vi "DDS_Clock.vi"() -> ()   [LabVIEW 2016] (continued)
dcp wait:1h:\rdcp wait::DROVER\rdcp 0 spi:DRL=0x4DD2F1AA4DC5D639\rdcp 0 spi:DRSS=0x1E1FFFFFFFF\rdcp 0 spi:DRR=0x70000\rdcp 0 update:+d\rdcp 0 update:-d\rdcp wait:1h:\rdcp wait::DROVER\rdcp 0 spi:DRL=0x4DC5D6394DB8BAC7\rdcp 0 spi:DRSS=0x1E1FFFFFFFF\rdcp 0 spi:DRR=0x70000\rdcp 0 update:+d\rdcp 0 update:-d\rdcp wait:1h:\rdcp wait::DROVER\rdcp 0 spi:DRL=0x4DB8BAC74DAB9F56\rdcp 0 spi:DRSS=0x1E1FFFFFFFF\rdcp 0 spi:DRR=0x70000\rdcp 0 update:+d\rdcp 0 update:-d\rdcp wait:1h:\rdcp wait::DROVER\rdcp 0 spi:DRL=0x4DAB9F564D9E83E4\rdcp 0 spi:DRSS=0x1E1FFFFFFFF\rdcp 0 spi:DRR=0x70000\rdcp 0 update:+d\rdcp 0 update:-d\rdcp wait:1h:\rdcp wait::DROVER\rdcp 0 spi:DRL=0x4D9E83E44D916873\rdcp 0 spi:DRSS=0x1E1FFFFFFFF\rdcp 0 spi:DRR=0x70000\rdcp 0 update:+d\rdcp 0 update:-d\rdcp wait:1h:\rdcp wait::DROVER\rdcp 0 spi:DRL=0x4D9168734D844D01\rdcp 0 spi:DRSS=0x1E1FFFFFFFF\rdcp 0 spi:DRR=0x70000\rdcp 0 update:+d\rdcp 0 update:-d\rdcp wait:1h:\rdcp wait::DROVER\rdcp 0 spi:DRL=0x4D844D014D773190\rdcp 0 spi:DRSS=0x1E1FFFFFFFF\rdcp 0 spi:DRR=0x70000\rdcp 0 update:+d\rdcp 0 update:-d\rdcp wait:1h:\rdcp wait::DROVER\rdcp 0 spi:DRL=0x4D7731904D6A161E\rdcp 0 spi:DRSS=0x1E1FFFFFFFF\rdcp 0 spi:DRR=0x70000\rdcp 0 update:+d\rdcp 0 update:-d\rdcp wait:1h:\rdcp wait::DROVER\rdcp 0 spi:DRL=0x4D6A161E4D5CFAAD\rdcp 0 spi:DRSS=0x1E1FFFFFFFF\rdcp 0 spi:DRR=0x70000\rdcp 0 update:+d\rdcp 0 update:-d\rdcp wait:1h:\rdcp wait::DROVER\rdcp 0 spi:DRL=0x4D5CFAAD4D4FDF3B\rdcp 0 spi:DRSS=0x1E1FFFFFFFF\rdcp 0 spi:DRR=0x70000\rdcp 0 update:+d\rdcp 0 update:-d\rdcp wait:1h:\rdcp wait::DROVER\rdcp 0 spi:DRL=0x4D4FDF3B4D42C3CA\rdcp 0 spi:DRSS=0x1E1FFFFFFFF\rdcp 0 spi:DRR=0x70000\rdcp 0 update:+d\rdcp 0 update:-d\rdcp wait:1h:\rdcp wait::DROVER\rdcp 0 spi:DRL=0x4D42C3CA4D35A858\rdcp 0 spi:DRSS=0x1E1FFFFFFFF\rdcp 0 spi:DRR=0x70000\rdcp 0 update:+d\rdcp 0 update:-d\rdcp wait:1h:\rdcp wait::DROVER\rdcp 0 spi:DRL=0x4D35A8584D288CE7\rdcp 0 spi:DRSS=0x1E1FFFFFFFF\rdcp 0 spi:DRR=0x70000\rdcp 0 update:+d\rdcp 0 update:-d\rdcp wait:1h:\rdcp wait::DROVER\rdcp 0 spi:DRL=0x4D288CE74D1B7176\rdcp 0 spi:DRSS=0x1E1FFFFFFFF\rdcp 0 spi:DRR=0x70000\rdcp 0 update:+d\rdcp 0 update:-d\rdcp wait:1h:\rdcp wait::DROVER\rdcp 0 spi:DRL=0x4D1B71764D0E5604\rdcp 0 spi:DRSS=0x1E1FFFFFFFF\rdcp 0 spi:DRR=0x70000\rdcp 0 update:+d\rdcp 0 update:-d\rdcp wait:1h:\rdcp wait::DROVER\rdcp 0 spi:DRL=0x4D0E56044D013A93\rdcp 0 spi:DRSS=0x1E1FFFFFFFF\rdcp 0 spi:DRR=0x70000\rdcp 0 update:+d\rdcp 0 update:-d\rdcp wait:1h:\rdcp wait::DROVER\rdcp 0 spi:DRL=0x4D013A934CF41F21\rdcp 0 spi:DRSS=0x1E1FFFFFFFF\rdcp 0 spi:DRR=0x70000\rdcp 0 update:+d\rdcp 0 update:-d\rdcp wait:1h:\rdcp wait::DROVER\rdcp 0 spi:DRL=0x4CF41F214CE703B0\rdcp 0 spi:DRSS=0x1E1FFFFFFFF\rdcp 0 spi:DRR=0x70000\rdcp 0 update:+d\rdcp 0 update:-d\rdcp wait:1h:\rdcp wait::DROVER\rdcp 0 spi:DRL=0x4CE703B04CD9E83E\rdcp 0 spi:DRSS=0x1E1FFFFFFFF\rdcp 0 spi:DRR=0x70000\rdcp 0 update:+d\rdcp 0 update:-d\rdcp wait:1h:\rdcp wait::DROVER\rdcp 0 spi:DRL=0x4CD9E83E4CCCCCCD\rdcp 0 spi:DRSS=0x1E1FFFFFFFF\rdcp 0 spi:DRR=0x70000\rdcp 0 update:+d\rdcp 0 update:-d\rdcp wait:1h:\rdcp wait::DROVER\rdcp 0 spi:DRL=0x4CD9E83E4CCCCCCD\rdcp 0 spi:DRSS=0xFFFFFFFF000001E1\rdcp 0 spi:DRR=0x7\rdcp 0 update:-d\rdcp 0 update:+d\rdcp wait:1h:\rdcp wait::DROVER\rdcp 0 spi:DRL=0x4CE703B04CD9E83E\rdcp 0 spi:DRSS=0xFFFFFFFF000001E1\rdcp 0 spi:DRR=0x7\rdcp 0 update:-d\rdcp 0 update:+d\rdcp wait:1h:\rdcp wait::DROVER\rdcp 0 spi:DRL=0x4CF41F214CE703B0\rdcp 0 spi:DRSS=0xFFFFFFFF000001E1\rdcp 0 spi:DRR=0x7\rdcp 0 update:-d\rdcp 0 update:+d\rdcp wait:1h:\rdcp wait::DROVER\rdcp 0 spi:DRL=0x4D013A934CF41F21\rdcp 0 spi:DRSS=0xFFFFFFFF000001E1\rdcp 0 spi:DRR=0x7\rdcp 0 update:-d\rdcp 0 update:+d\rdcp wait:1h:\rdcp wait::DROVER\rdcp 0 spi:DRL=0x4D0E56044D013A93\rdcp 0 spi:DRSS=0xFFFFFFFF000001E1\rdcp 0 spi:DRR=0x7\rdcp 0 update:-d\rdcp 0 update:+d\rdcp wait:1h:\rdcp wait::DROVER\rdcp 0 spi:DRL=0x4D1B71764D0E5604\rdcp 0 spi:DRSS=0xFFFFFFFF000001E1\rdcp 0 spi:DRR=0x7\rdcp 0 update:-d\rdcp 0 update:+d\rdcp wait:1h:\rdcp wait::DROVER\rdcp 0 spi:DRL=0x4D288CE74D1B7176\rdcp 0 spi:DRSS=0xFFFFFFFF000001E1\rdcp 0 spi:DRR=0x7\rdcp 0 update:-d\rdcp 0 update:+d\rdcp wait:1h:\rdcp wait::DROVER\rdcp 0 spi:DRL=0x4D35A8584D288CE7\rdcp 0 spi:DRSS=0xFFFFFFFF000001E1\rdcp 0 spi:DRR=0x7\rdcp 0 update:-d\rdcp 0 update:+d\rdcp wait:1h:\rdcp wait::DROVER\rdcp 0 spi:DRL=0x4D42C3CA4D35A858\rdcp 0 spi:DRSS=0xFFFFFFFF000001E1\rdcp 0 spi:DRR=0x7\rdcp 0 update:-d\rdcp 0 update:+d\rdcp wait:1h:\rdcp wait::DROVER\rdcp 0 spi:DRL=0x4D4FDF3B4D42C3CA\rdcp 0 spi:DRSS=0xFFFFFFFF000001E1\rdcp 0 spi:DRR=0x7\rdcp 0 update:-d\rdcp 0 update:+d\rdcp wait:1h:\rdcp wait::DROVER\rdcp 0 spi:DRL=0x4D5CFAAD4D4FDF3B\rdcp 0 spi:DRSS=0xFFFFFFFF000001E1\rdcp 0 spi:DRR=0x7\rdcp 0 update:-d\rdcp 0 update:+d\rdcp wait:1h:\rdcp wait::DROVER\rdcp 0 spi:DRL=0x4D6A161E4D5CFAAD\rdcp 0 spi:DRSS=0xFFFFFFFF000001E1\rdcp 0 spi:DRR=0x7\rdcp 0 update:-d\rdcp 0 update:+d\rdcp wait:1h:\rdcp wait::DROVER\rdcp 0 spi:DRL=0x4D7731904D6A161E\rdcp 0 spi:DRSS=0xFFFFFFFF000001E1\rdcp 0 spi:DRR=0x7\rdcp 0 update:-d\rdcp 0 update:+d\rdcp wait:1h:\rdcp wait::DROVER\rdcp 0 spi:DRL=0x4D844D014D773190\rdcp 0 spi:DRSS=0xFFFFFFFF000001E1\rdcp 0 spi:DRR=0x7\rdcp 0 update:-d\rdcp 0 update:+d\rdcp wait:1h:\rdcp wait::DROVER\rdcp 0 spi:DRL=0x4D9168734D844D01\rdcp 0 spi:DRSS=0xFFFFFFFF000001E1\rdcp 0 spi:DRR=0x7\rdcp 0 update:-d\rdcp 0 update:+d\rdcp wait:1h:\rdcp wait::DROVER\rdcp 0 spi:DRL=0x4D9E83E44D916873\rdcp 0 spi:DRSS=0xFFFFFFFF000001E1\rdcp 0 spi:DRR=0x7\rdcp 0 update:-d\rdcp 0 update:+d\rdcp wait:1h:\rdcp wait::DROVER\rdcp 0 spi:DRL=0x4DAB9F564D9E83E4\rdcp 0 spi:DRSS=0xFFFFFFFF000001E1\rdcp 0 spi:DRR=0x7\rdcp 0 update:-d\rdcp 0 update:+d\rdcp wait:1h:\rdcp wait::DROVER\rdcp 0 spi:DRL=0x4DB8BAC74DAB9F56\rdcp 0 spi:DRSS=0xFFFFFFFF000001E1\rdcp 0 spi:DRR=0x7\rdcp 0 update:-d\rdcp 0 update:+d\rdcp wait:1h:\rdcp wait::DROVER\rdcp 0 spi:DRL=0x4DC5D6394DB8BAC7\rdcp 0 spi:DRSS=0xFFFFFFFF000001E1\rdcp 0 spi:DRR=0x7\rdcp 0 update:-d\rdcp 0 update:+d\rdcp wait:1h:\rdcp wait::DROVER\rdcp 0 spi:DRL=0x4DD2F1AA4DC5D639\rdcp 0 spi:DRSS=0xFFFFFFFF000001E1\rdcp 0 spi:DRR=0x7\rdcp 0 update:-d\rdcp 0 update:+d\rdcp wait:1h:\rdcp wait::DROVER\rdcp 0 spi:DRL=0x4DE00D1B4DD2F1AA\rdcp 0 spi:DRSS=0xFFFFFFFF000001E1\rdcp 0 spi:DRR=0x7\rdcp 0 update:-d\rdcp 0 update:+d\rdcp wait:1h:\rdcp wait::DROVER\rdcp 0 spi:DRL=0x4DED288D4DE00D1B\rdcp 0 spi:DRSS=0xFFFFFFFF000001E1\rdcp 0 spi:DRR=0x7\rdcp 0 update:-d\rdcp 0 update:+d\rdcp wait:1h:\rdcp wait::DROVER\rdcp 0 spi:DRL=0x4DFA43FE4DED288D\rdcp 0 spi:DRSS=0xFFFFFFFF000001E1\rdcp 0 spi:DRR=0x7\rdcp 0 update:-d\rdcp 0 update:+d\rdcp wait:1h:\rdcp wait::DROVER\rdcp 0 spi:DRL=0x4E075F704DFA43FE\rdcp 0 spi:DRSS=0xFFFFFFFF000001E1\rdcp 0 spi:DRR=0x7\rdcp 0 update:-d\rdcp 0 update:+d\rdcp wait:1h:\rdcp wait::DROVER\rdcp 0 spi:DRL=0x4E147AE14E075F70\rdcp 0 spi:DRSS=0xFFFFFFFF000001E1\rdcp 0 spi:DRR=0x7\rdcp 0 update:-d\rdcp 0 update:+d\rdcp wait:1h:\rdcp wait::DROVER\rdcp 0 spi:DRL=0x4E2196534E147AE1\rdcp 0 spi:DRSS=0xFFFFFFFF000001E1\rdcp 0 spi:DRR=0x7\rdcp 0 update:-d\rdcp 0 update:+d\rdcp wait:1h:\rdcp wait::DROVER\rdcp 0 spi:DRL=0x4E2EB1C44E219653\rdcp 0 spi:DRSS=0xFFFFFFFF000001E1\rdcp 0 spi:DRR=0x7\rdcp 0 update:-d\rdcp 0 update:+d\rdcp wait:1h:\rdcp wait::DROVER\rdcp 0 spi:DRL=0x4E3BCD364E2EB1C4\rdcp 0 spi:DRSS=0xFFFFFFFF000001E1\rdcp 0 spi:DRR=0x7\rdcp 0 update:-d\rdcp 0 update:+d\rdcp wait:1h:\rdcp wait::DROVER\rdcp 0 spi:DRL=0x4E48E8A74E3BCD36\rdcp 0 spi:DRSS=0xFFFFFFFF000001E1\rdcp 0 spi:DRR=0x7\rdcp 0 update:-d\rdcp 0 update:+d\rdcp wait:1h:\rdcp wait::DROVER\rdcp 0 spi:DRL=0x4E5604194E48E8A7\rdcp 0 spi:DRSS=0xFFFFFFFF000001E1\rdcp 0 spi:DRR=0x7\rdcp 0 update:-d\rdcp 0 update:+d\rdcp wait:1h:\rdcp wait::DROVER\rdcp 0 spi:DRL=0x4E631F8A4E560419\rdcp 0 spi:DRSS=0xFFFFFFFF000001E1\rdcp 0 spi:DRR=0x7\rdcp 0 update:-d\rdcp 0 update:+d\rdcp wait:1h:\rdcp wait::DROVER\rdcp 0 spi:DRL=0x4E703AFB4E631F8A\rdcp 0 spi:DRSS=0xFFFFFFFF000001E1\rdcp 0 spi:DRR=0x7\rdcp 0 update:-d\rdcp 0 update:+d\rdcp wait:1h:\rdcp wait::DROVER\rdcp 0 spi:DRL=0x4E7D566D4E703AFB\rdcp 0 spi:DRSS=0xFFFFFFFF000001E1\rdcp 0 spi:DRR=0x7\rdcp 0 update:-d\rdcp 0 update:+d\rdcp wait:1h:\rdcp wait::DROVER\rdcp 0 spi:DRL=0x4E8A71DE4E7D566D\rdcp 0 spi:DRSS=0xFFFFFFFF000001E1\rdcp 0 spi:DRR=0x7\rdcp 0 update:-d\rdcp 0 update:+d\rdcp wait:1h:\rdcp wait::DROVER\rdcp 0 spi:DRL=0x4E978D504E8A71DE\rdcp 0 spi:DRSS=0xFFFFFFFF000001E1\rdcp 0 spi:DRR=0x7\rdcp 0 update:-d\rdcp 0 update:+d\rdcp wait:1h:\rdcp wait::DROVER\rdcp 0 spi:DRL=0x4EA4A8C14E978D50\rdcp 0 spi:DRSS=0xFFFFFFFF000001E1\rdcp 0 spi:DRR=0x7\rdcp 0 update:-d\rdcp 0 update:+d\rdcp wait:1h:\rdcp wait::DROVER\rdcp 0 spi:DRL=0x4EB1C4334EA4A8C1\rdcp 0 spi:DRSS=0xFFFFFFFF000001E1\rdcp 0 spi:DRR=0x7\rdcp 0 update:-d\rdcp 0 update:+d\rdcp wait:1h:\rdcp wait::DROVER\rdcp 0 spi:DRL=0x4EBEDFA44EB1C433\rdcp 0 spi:DRSS=0xFFFFFFFF000001E1\rdcp 0 spi:DRR=0x7\rdcp 0 update:-d\rdcp 0 update:+d\rdcp wait:1h:\rdcp wait::DROVER\rdcp 0 spi:DRL=0x4ECBFB164EBEDFA4\rdcp 0 spi:DRSS=0xFFFFFFFF000001E1\rdcp 0 spi:DRR=0x7\rdcp 0 update:-d\rdcp 0 update:+d\rdcp wait:1h:\rdcp wait::DROVER\rdcp 0 spi:DRL=0x4ED916874ECBFB16\rdcp 0 spi:DRSS=0xFFFFFFFF000001E1\rdcp 0 spi:DRR=0x7\rdcp 0 update:-d\rdcp 0 update:+d\rdcp wait:1h:\rdcp wait::DROVER\rdcp 0 spi:DRL=0x4EE631F94ED91687\rdcp 0 spi:DRSS=0xFFFFFFFF000001E1\rdcp 0 spi:DRR=0x7\rdcp 0 update:-d\rdcp 0 update:+d\rdcp wait:1h:\rdcp wait::DROVER\rdcp 0 spi:DRL=0x4EF34D6A4EE631F9\rdcp 0 spi:DRSS=0xFFFFFFFF000001E1\rdcp 0 spi:DRR=0x7\rdcp 0 update:-d\rdcp 0 update:+d\rdcp wait:1h:\rdcp wait::DROVER\rdcp 0 spi:DRL=0x4F0068DC4EF34D6A\rdcp 0 spi:DRSS=0xFFFFFFFF000001E1\rdcp 0 spi:DRR=0x7\rdcp 0 update:-d\rdcp 0 update:+d\rdcp wait:1h:\rdcp wait::DROVER\rdcp 0 spi:DRL=0x4F0D844D4F0068DC\rdcp 0 spi:DRSS=0xFFFFFFFF000001E1\rdcp 0 spi:DRR=0x7\rdcp 0 update:-d\rdcp 0 update:+d\rdcp wait:1h:\rdcp wait::DROVER\rdcp 0 spi:DRL=0x4F1A9FBE4F0D844D\rdcp 0 spi:DRSS=0xFFFFFFFF000001E1\rdcp 0 spi:DRR=0x7\rdcp 0 update:-d\rdcp 0 update:+d\rdcp wait:1h:\rdcp wait::DROVER\rdcp 0 spi:DRL=0x4F27BB304F1A9FBE\rdcp 0 spi:DRSS=0xFFFFFFFF000001E1\rdcp 0 spi:DRR=0x7\rdcp 0 update:-d\rdcp 0 update:+d\rdcp wait:1h:\rdcp wait::DROVER\rdcp 0 spi:DRL=0x4F34D6A14F27BB30\rdcp 0 spi:DRSS=0xFFFFFFFF000001E1\rdcp 0 spi:DRR=0x7\rdcp 0 update:-d\rdcp 0 update:+d\rdcp wait:1h:\rdcp wait::DROVER\rdcp 0 spi:DRL=0x4F41F2134F34D6A1\rdcp 0 spi:DRSS=0xFFFFFFFF000001E1\rdcp 0 spi:DRR=0x7\rdcp 0 update:-d\rdcp 0 update:+d\rdcp wait:1h:\rdcp wait::DROVER\rdcp 0 spi:DRL=0x4F4F0D844F41F213\rdcp 0 spi:DRSS=0xFFFFFFFF000001E1\rdcp 0 spi:DRR=0x7\rdcp 0 update:-d\rdcp 0 update:+d\rdcp wait:1h:\rdcp wait::DROVER\rdcp 0 spi:DRL=0x4F5C28F64F4F0D84\rdcp 0 spi:DRSS=0xFFFFFFFF000001E1\rdcp 0 spi:DRR=0x7\rdcp 0 update:-d\rdcp 0 update:+d\rdcp wait:1h:\rdcp wait::DROVER\rdcp 0 spi:DRL=0x4F6944674F5C28F6\rdcp 0 spi:DRSS=0xFFFFFFFF000001E1\rdcp 0 spi:DRR=0x7\rdcp 0 update:-d\rdcp 0 update:+d\rdcp wait:1h:\rdcp wait::DROVER\rdcp 0 spi:DRL=0x4F765FD94F694467\rdcp 0 spi:DRSS=0xFFFFFFFF000001E1\rdcp 0 spi:DRR=0x7\rdcp 0 update:-d\rdcp 0 update:+d\rdcp wait:1h:\rdcp wait::DROVER\rdcp 0 spi:DRL=0x4F837B4A4F765FD9\rdcp 0 spi:DRSS=0xFFFFFFFF000001E1\rdcp 0 spi:DRR=0x7\rdcp 0 update:-d\rdcp 0 update:+d\rdcp wait:1h:\rdcp wait::DROVER\rdcp 0 spi:DRL=0x4F9096BC4F837B4A\rdcp 0 spi:DRSS=0xFFFFFFFF000001E1\rdcp 0 spi:DRR=0x7\rdcp 0 update:-d\rdcp 0 update:+d\rdcp wait:1h:\rdcp wait::DROVER\rdcp 0 spi:DRL=0x4F9DB22D4F9096BC\rdcp 0 spi:DRSS=0xFFFFFFFF000001E1\rdcp 0 spi:DRR=0x7\rdcp 0 update:-d\rdcp 0 update:+d\rdcp wait:1h:\rdcp wait::DROVER\rdcp 0 spi:DRL=0x4FAACD9F4F9DB22D\rdcp 0 spi:DRSS=0xFFFFFFFF000001E1\rdcp 0 spi:DRR=0x7\rdcp 0 update:-d\rdcp 0 update:+d\rdcp wait:1h:\rdcp wait::DROVER\rdcp 0 spi:DRL=0x4FB7E9104FAACD9F\rdcp 0 spi:DRSS=0xFFFFFFFF000001E1\rdcp 0 spi:DRR=0x7\rdcp 0 update:-d\rdcp 0 update:+d\rdcp wait:1h:\rdcp wait::DROVER\rdcp 0 spi:DRL=0x4FC504814FB7E910\rdcp 0 spi:DRSS=0xFFFFFFFF000001E1\rdcp 0 spi:DRR=0x7\rdcp 0 update:-d\rdcp 0 update:+d\rdcp wait:1h:\rdcp wait::DROVER\rdcp 0 spi:DRL=0x4FD21FF34FC50481\rdcp 0 spi:DRSS=0xFFFFFFFF000001E1\rdcp 0 spi:DRR=0x7\rdcp 0 update:-d\rdcp 0 update:+d\rdcp wait:1h:\rdcp wait::DROVER\rdcp 0 spi:DRL=0x4FDF3B644FD21FF3\rdcp 0 spi:DRSS=0xFFFFFFFF000001E1\rdcp 0 spi:DRR=0x7\rdcp 0 update:-d\rdcp 0 update:+d\rdcp wait:1h:\rdcp wait::DROVER\rdcp 0 spi:DRL=0x4FEC56D64FDF3B64\rdcp 0 spi:DRSS=0xFFFFFFFF000001E1\rdcp 0 spi:DRR=0x7\rdcp 0 update:-d\rdcp 0 update:+d\rdcp wait:1h:\rdcp wait::DROVER\rdcp 0 spi:DRL=0x4FF972474FEC56D6\rdcp 0 spi:DRSS=0xFFFFFFFF000001E1\rdcp 0 spi:DRR=0x7\rdcp 0 update:-d\rdcp 0 update:+d\rdcp wait:1h:\rdcp wait::DROVER\rdcp 0 spi:DRL=0x50068DB94FF97247\rdcp 0 spi:DRSS=0xFFFFFFFF000001E1\rdcp 0 spi:DRR=0x7\rdcp 0 update:-d\rdcp 0 update:+d\rdcp wait:1h:\rdcp wait::DROVER\rdcp 0 spi:DRL=0x5013A92A50068DB9\rdcp 0 spi:DRSS=0xFFFFFFFF000001E1\rdcp 0 spi:DRR=0x7\rdcp 0 update:-d\rdcp 0 update:+d\rdcp wait:1h:\rdcp wait::DROVER\rdcp 0 spi:DRL=0x5020C49C5013A92A\rdcp 0 spi:DRSS=0xFFFFFFFF000001E1\rdcp 0 spi:DRR=0x7\rdcp 0 update:-d\rdcp 0 update:+d\rdcp wait:1h:\rdcp wait::DROVER\rdcp 0 spi:DRL=0x502DE00D5020C49C\rdcp 0 spi:DRSS=0xFFFFFFFF000001E1\rdcp 0 spi:DRR=0x7\rdcp 0 update:-d\rdcp 0 update:+d\rdcp wait:1h:\rdcp wait::DROVER\rdcp 0 spi:DRL=0x503AFB7F502DE00D\rdcp 0 spi:DRSS=0xFFFFFFFF000001E1\rdcp 0 spi:DRR=0x7\rdcp 0 update:-d\rdcp 0 update:+d\rdcp wait:1h:\rdcp wait::DROVER\rdcp 0 spi:DRL=0x504816F0503AFB7F\rdcp 0 spi:DRSS=0xFFFFFFFF000001E1\rdcp 0 spi:DRR=0x7\rdcp 0 update:-d\rdcp 0 update:+d\rdcp wait:1h:\rdcp wait::DROVER\rdcp 0 spi:DRL=0x50553261504816F0\rdcp 0 spi:DRSS=0xFFFFFFFF000001E1\rdcp 0 spi:DRR=0x7\rdcp 0 update:-d\rdcp 0 update:+d\rdcp wait:1h:\rdcp wait::DROVER\rdcp 0 spi:DRL=0x50624DD350553261\rdcp 0 spi:DRSS=0xFFFFFFFF000001E1\rdcp 0 spi:DRR=0x7\rdcp 0 update:-d\rdcp 0 update:+d\rdcp wait:1h:\rdcp wait::DROVER\rdcp 0 spi:DRL=0x506F694450624DD3\rdcp 0 spi:DRSS=0xFFFFFFFF000001E1\rdcp 0 spi:DRR=0x7\rdcp 0 update:-d\rdcp 0 update:+d\rdcp wait:1h:\rdcp wait::DROVER\rdcp 0 spi:DRL=0x507C84B6506F6944\rdcp 0 spi:DRSS=0xFFFFFFFF000001E1\rdcp 0 spi:DRR=0x7\rdcp 0 update:-d\rdcp 0 update:+d\rdcp wait:1h:\rdcp wait::DROVER\rdcp 0 spi:DRL=0x5089A027507C84B6\rdcp 0 spi:DRSS=0xFFFFFFFF000001E1\rdcp 0 spi:DRR=0x7\rdcp 0 update:-d\rdcp 0 update:+d\rdcp wait:1h:\rdcp wait::DROVER\rdcp 0 spi:DRL=0x5096BB995089A027\rdcp 0 spi:DRSS=0xFFFFFFFF000001E1\rdcp 0 spi:DRR=0x7\rdcp 0 update:-d\rdcp 0 update:+d\rdcp wait:1h:\rdcp wait::DROVER\rdcp 0 spi:DRL=0x50A3D70A5096BB99\rdcp 0 spi:DRSS=0xFFFFFFFF000001E1\rdcp 0 spi:DRR=0x7\rdcp 0 update:-d\rdcp 0 update:+d\rdcp wait:1h:\rdcp wait::DROVER\rdcp 0 spi:DRL=0x50B0F27C50A3D70A\rdcp 0 spi:DRSS=0xFFFFFFFF000001E1\rdcp 0 spi:DRR=0x7\rdcp 0 update:-d\rdcp 0 update:+d\rdcp wait:1h:\rdcp wait::DROVER\rdcp 0 spi:DRL=0x50BE0DED50B0F27C\rdcp 0 spi:DRSS=0xFFFFFFFF000001E1\rdcp 0 spi:DRR=0x7\rdcp 0 update:-d\rdcp 0 update:+d\rdcp wait:1h:\rdcp wait::DROVER\rdcp 0 spi:DRL=0x50CB295F50BE0DED\rdcp 0 spi:DRSS=0xFFFFFFFF000001E1\rdcp 0 spi:DRR=0x7\rdcp 0 update:-d\rdcp 0 update:+d\rdcp wait:1h:\rdcp wait::DROVER\rdcp 0 spi:DRL=0x50D844D050CB295F\rdcp 0 spi:DRSS=0xFFFFFFFF000001E1\rdcp 0 spi:DRR=0x7\rdcp 0 update:-d\rdcp 0 update:+d\rdcp wait:1h:\rdcp wait::DROVER\rdcp 0 spi:DRL=0x50E5604250D844D0\rdcp 0 spi:DRSS=0xFFFFFFFF000001E1\rdcp 0 spi:DRR=0x7\rdcp 0 update:-d\rdcp 0 update:+d\rdcp wait:1h:\rdcp wait::DROVER\rdcp 0 spi:DRL=0x50F27BB350E56042\rdcp 0 spi:DRSS=0xFFFFFFFF000001E1\rdcp 0 spi:DRR=0x7\rdcp 0 update:-d\rdcp 0 update:+d\rdcp wait:1h:\rdcp wait::DROVER\rdcp 0 spi:DRL=0x50FF972450F27BB3\rdcp 0 spi:DRSS=0xFFFFFFFF000001E1\rdcp 0 spi:DRR=0x7\rdcp 0 update:-d\rdcp 0 update:+d\rdcp wait:1h:\rdcp wait::DROVER\rdcp 0 spi:DRL=0x510CB29650FF9724\rdcp 0 spi:DRSS=0xFFFFFFFF000001E1\rdcp 0 spi:DRR=0x7\rdcp 0 update:-d\rdcp 0 update:+d\rdcp wait:1h:\rdcp wait::DROVER\rdcp 0 spi:DRL=0x5119CE07510CB296\rdcp 0 spi:DRSS=0xFFFFFFFF000001E1\rdcp 0 spi:DRR=0x7\rdcp 0 update:-d\rdcp 0 update:+d\rdcp wait:1h:\rdcp wait::DROVER\rdcp 0 spi:DRL=0x5126E9795119CE07\rdcp 0 spi:DRSS=0xFFFFFFFF000001E1\rdcp 0 spi:DRR=0x7\rdcp 0 update:-d\rdcp 0 update:+d\rdcp wait:1h:\rdcp wait::DROVER\rdcp 0 spi:DRL=0x513404EA5126E979\rdcp 0 spi:DRSS=0xFFFFFFFF000001E1\rdcp 0 spi:DRR=0x7\rdcp 0 update:-d\rdcp 0 update:+d\rdcp wait:1h:\rdcp wait::DROVER\rdcp 0 spi:DRL=0x5141205C513404EA\rdcp 0 spi:DRSS=0xFFFFFFFF000001E1\rdcp 0 spi:DRR=0x7\rdcp 0 update:-d\rdcp 0 update:+d\rdcp wait:1h:\rdcp wait::DROVER\rdcp 0 spi:DRL=0x514E3BCD5141205C\rdcp 0 spi:DRSS=0xFFFFFFFF000001E1\rdcp 0 spi:DRR=0x7\rdcp 0 update:-d\rdcp 0 update:+d\rdcp wait:1h:\rdcp wait::DROVER\rdcp 0 spi:DRL=0x515B573F514E3BCD\rdcp 0 spi:DRSS=0xFFFFFFFF000001E1\rdcp 0 spi:DRR=0x7\rdcp 0 update:-d\rdcp 0 update:+d\rdcp wait:1h:\rdcp wait::DROVER\rdcp 0 spi:DRL=0x516872B0515B573F\rdcp 0 spi:DRSS=0xFFFFFFFF000001E1\rdcp 0 spi:DRR=0x7\rdcp 0 update:-d\rdcp 0 update:+d\rdcp wait:1h:\rdcp wait::DROVER\rdcp 0 spi:DRL=0x51758E22516872B0\rdcp 0 spi:DRSS=0xFFFFFFFF000001E1\rdcp 0 spi:DRR=0x7\rdcp 0 update:-d\rdcp 0 update:+d\rdcp wait:1h:\rdcp wait::DROVER\rdcp 0 spi:DRL=0x5182A99351758E22\rdcp 0 spi:DRSS=0xFFFFFFFF000001E1\rdcp 0 spi:DRR=0x7\rdcp 0 update:-d\rdcp 0 update:+d\rdcp wait:1h:\rdcp wait::DROVER\rdcp 0 spi:DRL=0x518FC5055182A993\rdcp 0 spi:DRSS=0xFFFFFFFF000001E1\rdcp 0 spi:DRR=0x7\rdcp 0 update:-d\rdcp 0 update:+d\rdcp wait:1h:\rdcp wait::DROVER\rdcp 0 spi:DRL=0x519CE076518FC505\rdcp 0 spi:DRSS=0xFFFFFFFF000001E1\rdcp 0 spi:DRR=0x7\rdcp 0 update:-d\rdcp 0 update:+d\rdcp wait:1h:\rdcp wait::DROVER\rdcp 0 spi:DRL=0x51A9FBE7519CE076\rdcp 0 spi:DRSS=0xFFFFFFFF000001E1\rdcp 0 spi:DRR=0x7\rdcp 0 update:-d\rdcp 0 update:+d\rdcp wait:1h:\rdcp wait::DROVER\rdcp 0 spi:DRL=0x51B7175951A9FBE7\rdcp 0 spi:DRSS=0xFFFFFFFF000001E1\rdcp 0 spi:DRR=0x7\rdcp 0 update:-d\rdcp 0 update:+d\rdcp wait:1h:\rdcp wait::DROVER\rdcp 0 spi:DRL=0x51C432CA51B71759\rdcp 0 spi:DRSS=0xFFFFFFFF000001E1\rdcp 0 spi:DRR=0x7\rdcp 0 update:-d\rdcp 0 update:+d\rdcp wait:1h:\rdcp wait::DROVER\rdcp 0 spi:DRL=0x51D14E3C51C432CA\rdcp 0 spi:DRSS=0xFFFFFFFF000001E1\rdcp 0 spi:DRR=0x7\rdcp 0 update:-d\rdcp 0 update:+d\rdcp wait:1h:\rdcp wait::DROVER\rdcp 0 spi:DRL=0x51DE69AD51D14E3C\rdcp 0 spi:DRSS=0xFFFFFFFF000001E1\rdcp 0 spi:DRR=0x7\rdcp 0 update:-d\rdcp 0 update:+d\rdcp wait:1h:\rdcp wait::DROVER\rdcp 0 spi:DRL=0x51EB851F51DE69AD\rdcp 0 spi:DRSS=0xFFFFFFFF000001E1\rdcp 0 spi:DRR=0x7\rdcp 0 update:-d\rdcp 0 update:+d\rdcp wait:1h:\rdcp wait::DROVER\rdcp 0 spi:DRL=0x51EB851F51DE69AD\rdcp 0 spi:DRSS=0x1E1FFFFFFFF\rdcp 0 spi:DRR=0x70000\rdcp 0 update:+d\rdcp 0 update:-d\rdcp wait:1h:\rdcp wait::DROVER\rdcp 0 spi:DRL=0x51DE69AD51D14E3C\rdcp 0 spi:DRSS=0x1E1FFFFFFFF\rdcp 0 spi:DRR=0x70000\rdcp 0 update:+d\rdcp 0 update:-d\rdcp wait:1h:\rdcp wait::DROVER\rdcp 0 spi:DRL=0x51D14E3C51C432CA\rdcp 0 spi:DRSS=0x1E1FFFFFFFF\rdcp 0 spi:DRR=0x70000\rdcp 0 update:+d\rdcp 0 update:-d\rdcp wait:1h:\rdcp wait::DROVER\rdcp 0 spi:DRL=0x51C432CA51B71759\rdcp 0 spi:DRSS=0x1E1FFFFFFFF\rdcp 0 spi:DRR=0x70000\rdcp 0 update:+d\rdcp 0 update:-d\rdcp wait:1h:\rdcp wait::DROVER\rdcp 0 spi:DRL=0x51B7175951A9FBE7\rdcp 0 spi:DRSS=0x1E1FFFFFFFF\rdcp 0 spi:DRR=0x70000\rdcp 0 update:+d\rdcp 0 update:-d\rdcp wait:1h:\rdcp wait::DROVER\rdcp 0 spi:DRL=0x51A9FBE7519CE076\rdcp 0 spi:DRSS=0x1E1FFFFFFFF\rdcp 0 spi:DRR=0x70000\rdcp 0 update:+d\rdcp 0 update:-d\rdcp wait:1h:\rdcp wait::DROVER\rdcp 0 spi:DRL=0x519CE076518FC505\rdcp 0 spi:DRSS=0x1E1FFFFFFFF\rdcp 0 spi:DRR=0x70000\rdcp 0 update:+d\rdcp 0 update:-d\rdcp wait:1h:\rdcp wait::DROVER\rdcp 0 spi:DRL=0x518FC5055182A993\rdcp 0 spi:DRSS=0x1E1FFFFFFFF\rdcp 0 spi:DRR=0x70000\rdcp 0 update:+d\rdcp 0 update:-d\rdcp wait:1h:\rdcp wait::DROVER\rdcp 0 spi:DRL=0x5182A99351758E22\rdcp 0 spi:DRSS=0x1E1FFFFFFFF\rdcp 0 spi:DRR=0x70000\rdcp 0 update:+d\rdcp 0 update:-d\rdcp wait:1h:\rdcp wait::DROVER\rdcp 0 spi:DRL=0x51758E22516872B0\rdcp 0 spi:DRSS=0x1E1FFFFFFFF\rdcp 0 spi:DRR=0x70000\rdcp 0 update:+d\rdcp 0 update:-d\rdcp wait:1h:\r
